vi "Restore Configuration.vi"(8 "error in (no error)":errorcluster, 10 "File path":path, 11 "Monitor-Pulse in":refnum<class "Monitor-Pulse.lvclass">) -> (0 "error out":errorcluster, 1 "Section out":string, 2 "File path out":path, 3 "Monitor-Pulse out":refnum<class "Monitor-Pulse.lvclass">)   [LabVIEW 2016, in "Monitor-Pulse.lvclass"]
uses:
  Monitor-Pulse.lvclass
  Monitor-Pulse.lvclass/Monitor-Pulse.ctl
  <vilib>/Utility/error.llb/Error Cluster From Error Code.vi
  <vilib>/ErrorRing/Error Ring.xnode
  Controllers/Application Controller/Application Controller.lvclass
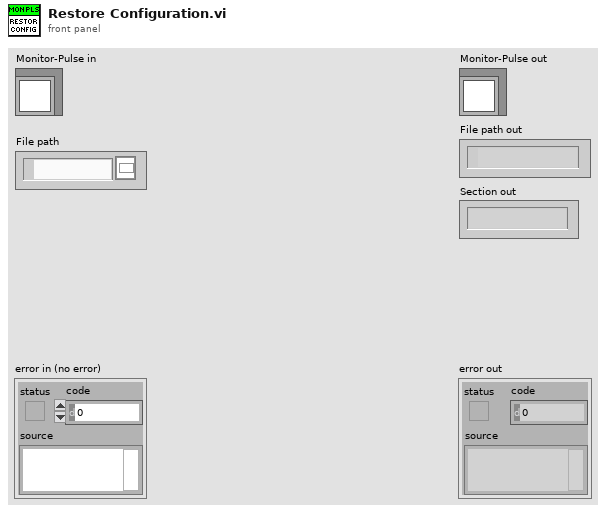
[diagram p1: front panel]
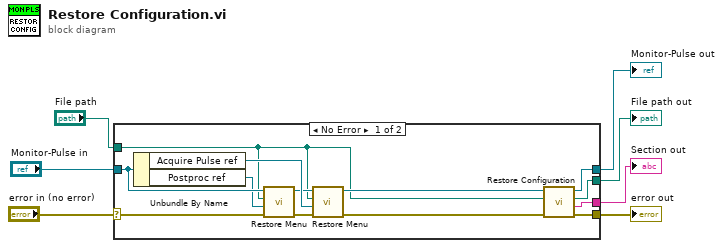
[diagram p0: block diagram]
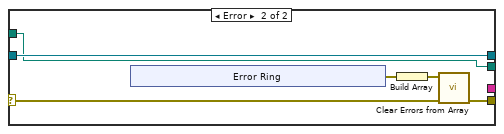
[diagram p2: hidden frame]
diagram:
  n1 = case shown="No Error" "error in (no error)" {
    selector: "error in (no error)" -> [w8 w22]
    tunnel: [w20 _] -> w7
    tunnel: [w19 w26] -> w6
    tunnel: "Monitor-Pulse in" -> [w18 w26]
    tunnel: [w17 w21] -> w4
    tunnel: [w16 w25] -> w3
    tunnel: "File path" -> [w9 w25]
    frame No Error {
      n2 = Unbundle By Name(w18) -> ("Acquire Pulse ref"=w13:refnum<vi>, "Postproc ref"=w10:refnum<vi>)
      n3 = call-dynamic "Restore Menu.vi"("error in (no error)"=w8, "Menu ref"=w10, "File path"=w9, "Monitor-Pulse in"=w18) -> ("error out"=w11:errorcluster, "Monitor-Pulse out"=w12:refnum<class "Monitor-Pulse.lvclass">)  [unwired: 4 in, 2 out]
      n4 = call-dynamic "Restore Menu.vi"("error in (no error)"=w11, "Menu ref"=w13, "File path"=w9, "Monitor-Pulse in"=w12) -> ("error out"=w14:errorcluster, "Monitor-Pulse out"=w15:refnum<class "Monitor-Pulse.lvclass">)  [unwired: 4 in, 2 out]
      n5 = call-parent "Restore Configuration.vi"("error in (no error)"=w14, "File path"=w9, "Measure Object in"=w15) -> ("error out"=w17:errorcluster, "Section out"=w20:string, "File path out"=w16:path, "Measure Object out"=w19:refnum<class "Monitor-Pulse.lvclass">)  [unwired: 5 in]
    }
    frame Error {
      n6 = xnode "Error Ring"() -> ("error out"=w24:errorcluster)
      n7 = Build Array(w24) -> (w23:errorcluster[])
      n8 = call "Clear Errors from Array.vi"("Error In"=w22, "Errors to clear"=w23) -> ("Error Out"=w21:errorcluster)  [unwired: 8 in, 1 out]
    }
  }
  "error out" <- w4
  "Monitor-Pulse out" <- w6
  "File path out" <- w3
  "Section out" <- w7
